vi "svfa_Rect Window Frequency Response.vi"(1 "N":i32, 2 "f":dbl format="%.2f") -> (0 "H(f)":cdb format="%.2f")   [LabVIEW 2017]
panel:
  # "Frequency Response of Rect Window"
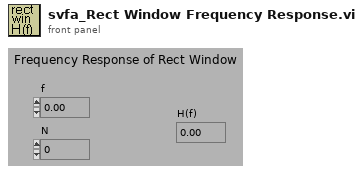
[diagram p1: front panel]
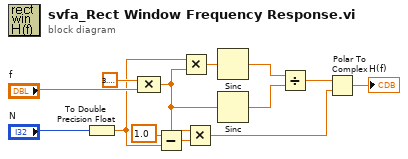
[diagram p0: block diagram]
diagram:
  n1 = To Double Precision Float(number="N") -> (double precision float=w1:dbl)
  n2 = Compound Arithmetic op=MULTIPLY(3.141592653589793 ("Pi"), "f") -> (w4:dbl)
  n3 = Subtract(x=1.0, y=w1) -> (x-y=w2:dbl)
  n4 = Multiply(x=w1, y=w4) -> (x*y=w7:dbl)
  n5 = Multiply(x=w4, y=w2) -> (x*y=w9:dbl)
  n6 = Sinc(1:w7) -> (0:w6:dbl)
  n7 = Sinc(1:w4) -> (0:w5:dbl)
  n8 = Divide(x=w6, y=w5) -> (x/y=w11:dbl)
  n9 = Polar To Complex(1:w9, 2:w11) -> (0:→"H(f)":cdb)
